vi "Result_Test.vi"(8 "error in (no error)":errorcluster caption="entrée d'erreur (pas d'erreur)", 11 "Delay en entrée":refnum<class "P2201_Scan_SN.lvclass">) -> (0 "error out":errorcluster caption="sortie d'erreur", 3 "Delay en sortie":refnum<class "P2201_Scan_SN.lvclass">)   [LabVIEW 2020, in "Library Test.lvlib" / "P2201_Scan_SN.lvclass"]
uses:
  P2201_Scan_SN.lvclass
  C:/Users/ngarcin/OneDrive - Altyor/Standard TB/Class/Test/Test (Default)/Test (Default).lvclass
  Test_Without_Instr/Test_Without_Inst.lvclass
  P2201_Scan_SN.lvclass/P2201_Scan_SN.ctl
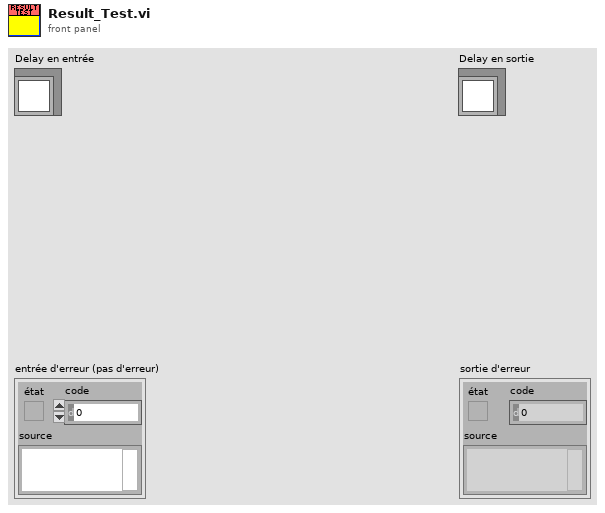
[diagram p1: front panel]
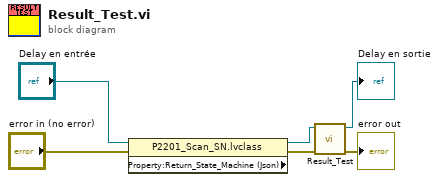
[diagram p0: block diagram]
diagram:
  n1 = property class="P2201_Scan_SN.lvclass" props=["Property:Return_State_Machine (Json)"](reference="Delay en entrée", error in="error in (no error)") -> (reference out=w3:refnum<class "P2201_Scan_SN.lvclass">, error out=w1:errorcluster)  [unwired: 1 out]
  n2 = call-parent "Result_Test.vi"("error in (no error)"=w1, "Test_Without_Inst en entrée"=w3) -> ("error out"=→"error out":errorcluster, "Test_Without_Inst en sortie"=→"Delay en sortie":refnum<class "P2201_Scan_SN.lvclass">)  [unwired: 8 in]
